vi "freq_to_wavelength.vi"(11 "frequency_hz":dbl) -> (3 "wavelength_m":dbl)   [LabVIEW 2025]
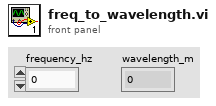
[diagram p1: front panel]
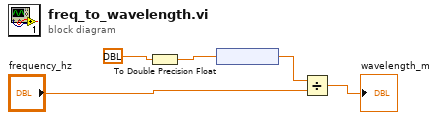
[diagram p0: block diagram]
diagram:
  n1 = To Double Precision Float(number=ext[unit] 299792458.0) -> (double precision float=w2:dbl[unit])
  n2 = node(w2) -> (w1:dbl)
  n3 = Divide(x=w1, y="frequency_hz") -> (x/y=→"wavelength_m":dbl)
